vi "Load from File.vi"(8 "error in (no error)":errorcluster, 10 "Path":path, 11 "GPack File in":refnum<class "GPack File.lvclass">) -> (0 "error out":errorcluster, 3 "GPack File out":refnum<class "GPack File.lvclass">)   [LabVIEW 2020, in "GPack.lvlib" / "GPack File.lvclass"]
uses:
  GPack File.lvclass
  File Contents.ctl
  Package Info.ctl
  Dependency.ctl
  GPack File.lvclass/GPack File.ctl
  48eed59b-c8a8-4acb-82a9-ed4313845678.vi
  <vilib>/JDP Science/JSONtext/JSON text to Variant.vi
  <vilib>/JDP Science/JSONtext/LVClass Serializer/JSONtext LVClass Serializer.lvclass
  GPack.lvlib
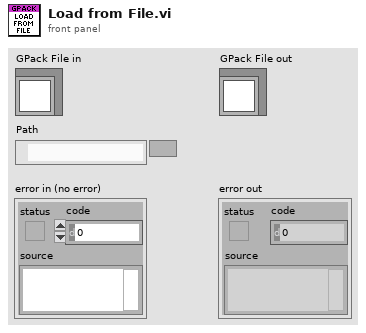
[diagram p1: front panel]
types:
  T1 = typedef "GPack.lvlib/GPack File.lvclass/File Contents.ctl" = cluster{"Info":T2, "Dependencies":T3[]}
  T2 = typedef "GPack.lvlib/Package Info.ctl" = cluster{"Name":string, "Type":string, "Host":string, "Path":string, "Branch":string, "Version":string}
  T3 = typedef "GPack.lvlib/Dependency.ctl" = cluster{"Info":T2, "Path":path}
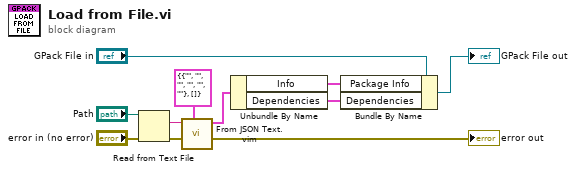
[diagram p0: block diagram]
diagram:
  n1 = Read from Text File(file (use dialog)="Path", error in="error in (no error)") -> (text=w8:string, error out=w7:errorcluster)  [unwired: 2 in, 2 out]
  n2 = call "From JSON Text.vim"("Data Type and Default Value"=T1 {"Info"={"Name"="", "Type"="", "Host"="", "Path"="", "Branch"="", "Version"=""}, "Dependencies"=[]} ("File Contents"), "error in (no error)"=w7, "JSON"=w8) -> ("error out"=→"error out":errorcluster, "Data out"=w5:T1)  [unwired: 7 in]
  n3 = Unbundle By Name(w5) -> ("Info"=w3:T2, "Dependencies"=w2:T3[])
  n4 = Bundle By Name(cluster="GPack File in", "Package Info"=w3, "Dependencies"=w2) -> (→"GPack File out":refnum<class "GPack File.lvclass">)
